vi "Test.vi"() -> ()   [LabVIEW 2015]
doc: "This VI is called when test mode begins, and will automatically be terminated when it ends. You can add manual or automatic tests and invoke them from the dashboard."
uses:
  Drive Base - Controlled Mode - TypeDef.ctl
  Drive Base Mode.ctl
panel:
  in  "notification":T1
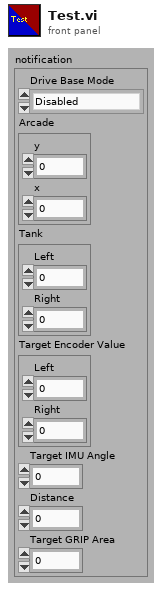
[diagram p1: front panel]
types:
  T1 = typedef "Drive Base - Controlled Mode - TypeDef.ctl" = cluster{"Drive Base Mode":T2, "Arcade":cluster{"y":dbl, "x":dbl}, "Tank":cluster{"Left":dbl, "Right":dbl}, "Target Encoder Value":cluster{"Left":dbl, "Right":dbl}, "Target IMU Angle":dbl, "Distance":dbl, "Target GRIP Area":dbl}
  T2 = typedef "Drive Base Mode.ctl" = enum16{"Disabled", "Controlled - Arcade", "Controlled - Tank", "Braked", "GRIP", "Encoder", "IMU", "Distance"}
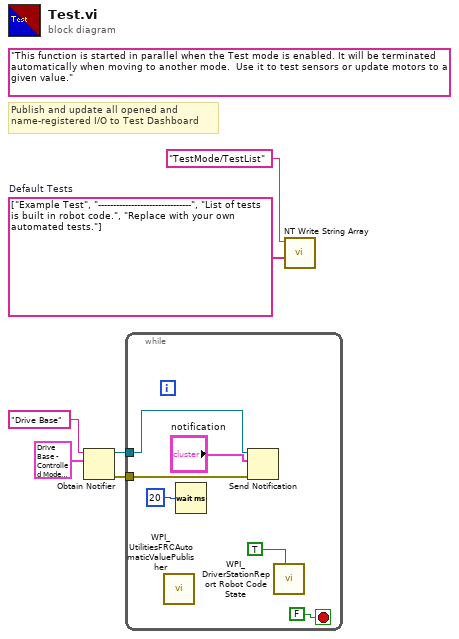
[diagram p0: block diagram]
diagram:
  w6 = string[] ["Example Test", "-------------------------------", "List of tests is built in robot code.", "Replace with your own automated tests."]  # Default Tests
  (unwired) "This function is started in parallel when the Test mode is enabled. It will be terminated automatically when moving to another mode.  Use it to test sensors or update motors to a given value."
  # "Publish and update all opened and\nname-registered I/O to Test Dashboard"
  n1 = Obtain Notifier(name (unnamed)="Drive Base", notification data type=T1 {"Drive Base Mode"=enum."Disabled", "Arcade"={"y"=0.0, "x"=0.0}, "Tank"={"Left"=0.0, "Right"=0.0}, "Target Encoder Value"={"Left"=0.0, "Right"=0.0}, "Target IMU Angle"=0.0, "Distance"=0.0, "Target GRIP Area"=0.0}) -> (notifier out=w2:refnum<notifier>, error out=w1:errorcluster)  [unwired: 2 in, 1 out]
  n2 = while {
    tunnel: w2 -> [w8]
    tunnel: w1 -> [w9]
    stop <- FALSE stop-if-true
    n3 = call <vilib>:"WPI_UtilitiesFRCAutomaticValuePublisher.vi"() -> ()  [unwired: 12 in]
    n4 = Wait (ms)(milliseconds to wait=u32 20) -> ()  [unwired: 1 out]
    n5 = Send Notification(notification="notification", notifier=w8, error in (no error)=w9) -> ()  [unwired: 2 out]
    n6 = call <vilib>:"WPI_DriverStationReport Robot Code State.vi"("Test"=TRUE ("Autonomous")) -> ()  [unwired: 10 in, 1 out]
  }
  n7 = call <vilib>:"NT Write String Array.vi"("String Array"=w6, "Name"="TestMode/TestList") -> ()  [unwired: 9 in, 1 out]
